vi "Calibration(Z).vi"(7 "Load calibration data":bool, 8 "error in (no error)":errorcluster, 9 "Save calibration data":bool, 10 "Done Button":bool, 11 "Acceleration [g]| Voltage [V]":dbl[][](array[numeric])=[[1.0, 2.02], [3.0, 3.3], [-3.0, 0.25], [0.0, 1.7]]) -> (0 "error out":errorcluster, 2 "Interpolation method":T1(ring), 3 "Distance [cm]| Voltage [V]":dbl[][](array[numeric])=[[1.0, 2.02], [3.0, 3.3], [-3.0, 0.25], [0.0, 1.7]])   [LabVIEW 2025]
uses:
  <vilib>/Utility/file.llb/Write To Spreadsheet File (DBL).vi
  <vilib>/Utility/file.llb/Read From Spreadsheet File (DBL).vi
  <vilib>/gmath/NI_Gmath.lvlib
panel:
  in  "method":T1(ring)=enum."linear"
  in  "Refresh Button":bool
  out "Transfer function":cluster{"yi":dbl[], "xi used":dbl[]}[](graph)=[{"yi"=[2.02, 3.3, 0.25, 1.7], "xi used"=[1.0, 3.0, -3.0, 0.0]}, {"yi"=[0.25, 0.2953125, 0.340625, 0.38593750000000004, 0.43125, 0.47656250000000006, 0.5218750000000001, 0.5671875000000001, 0.6125, 0.6578125, 0.703125, 0.7484375, 0.79375, 0.8390624999999999, 0.8843749999999999, 0.9296875, 0.975, 1.0203125, 1.065625, 1.1109375, 1.15625, 1.2015625, 1.246875, 1.2921874999999998, 1.3375, 1.3828125, 1.4281249999999999, 1.4734374999999997, 1.5187499999999998, 1.5640625, 1.609375, 1.6546875, 1.7, 1.71, 1.7199999999999998, 1.7299999999999998, 1.7399999999999998, 1.7499999999999998, 1.7599999999999998, 1.7699999999999998, 1.7799999999999998, 1.7899999999999998, 1.7999999999999998, 1.8099999999999998, 1.8199999999999998, 1.8299999999999998, 1.8399999999999999, 1.8499999999999999, 1.8599999999999999, 1.8699999999999999, 1.88, 1.89, 1.9, 1.91, 1.92, 1.93, 1.94, 1.95, 1.96, 1.97, 1.98, 1.99, 2.0, 2.01, 2.02, 2.0599999999999996, 2.0999999999999996, 2.1399999999999997, 2.1799999999999997, 2.2199999999999998, 2.26, 2.3, 2.34, 2.38, 2.42, 2.46, 2.5, 2.54, 2.58, 2.62, 2.66, 2.7, 2.74, 2.7800000000000002, 2.8200000000000003, 2.8600000000000003, 2.9000000000000004, 2.9400000000000004, 2.98, 3.0199999999999996, 3.0599999999999996, 3.0999999999999996, 3.1399999999999997, 3.1799999999999997, 3.2199999999999998, 3.26, 3.3], "xi used"=[-3.0, -2.90625, -2.8125, -2.71875, -2.625, -2.53125, -2.4375, -2.34375, -2.25, -2.15625, -2.0625, -1.96875, -1.8750000000000002, -1.7812500000000002, -1.6875000000000002, -1.59375, -1.5, -1.40625, -1.3125, -1.2187500000000004, -1.125, -1.0312499999999996, -0.9375, -0.8437500000000003, -0.75, -0.6562499999999998, -0.5625000000000002, -0.4687500000000006, -0.37500000000000033, -0.2812500000000001, -0.18749999999999983, -0.09374999999999958, 0.0, 0.03125000000000003, 0.06249999999999917, 0.0937499999999992, 0.12499999999999922, 0.15624999999999925, 0.18749999999999928, 0.2187499999999993, 0.24999999999999933, 0.28124999999999933, 0.3124999999999994, 0.34374999999999944, 0.37499999999999944, 0.40624999999999944, 0.4374999999999995, 0.46874999999999956, 0.49999999999999956, 0.5312499999999996, 0.5624999999999996, 0.5937499999999996, 0.6249999999999997, 0.6562499999999998, 0.6874999999999998, 0.7187499999999998, 0.7499999999999998, 0.7812499999999998, 0.8124999999999998, 0.8437499999999998, 0.8749999999999999, 0.90625, 0.9375, 0.9687499999999993, 1.0, 1.0625, 1.125, 1.1875, 1.25, 1.3125, 1.375, 1.4375, 1.5, 1.5625, 1.625, 1.6875, 1.75, 1.8125, 1.875, 1.9375, 2.0, 2.0625, 2.125, 2.1875, 2.25, 2.3125, 2.375, 2.4375, 2.5, 2.5625, 2.625, 2.6875, 2.75, 2.8125, 2.875, 2.9375, 3.0]}]
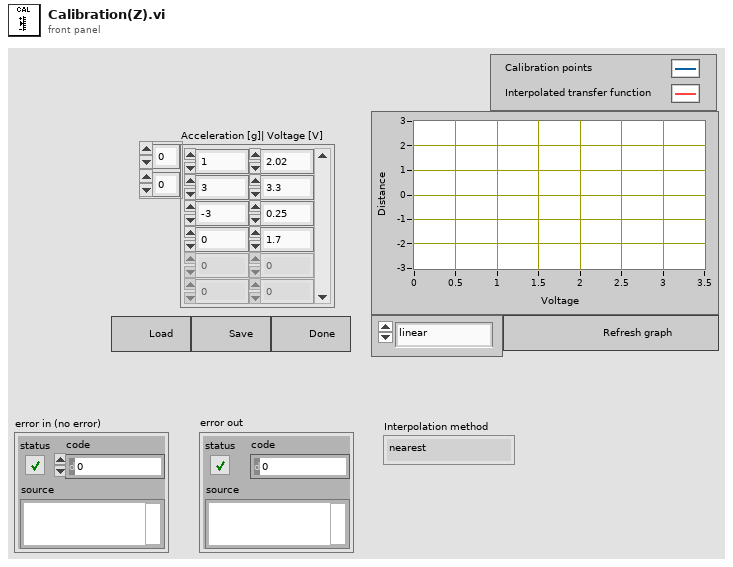
[diagram p1: front panel]
types:
  T1 = enum16{"nearest", "linear", "spline", "cubic Hermite", "Lagrange"}
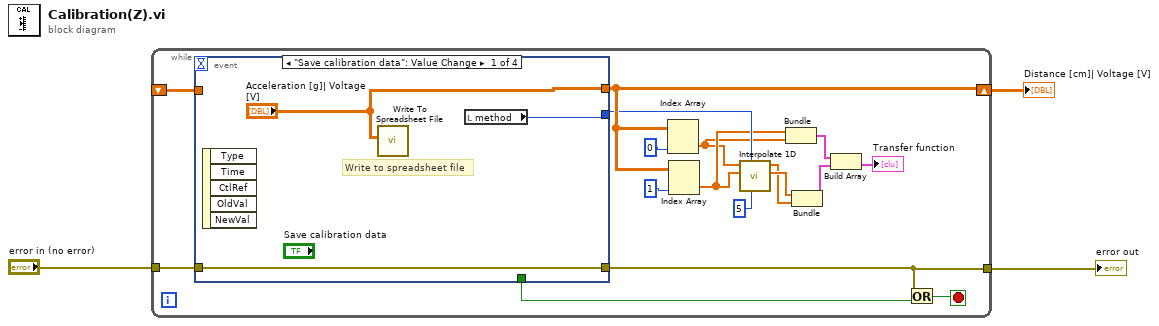
[diagram p0: block diagram]
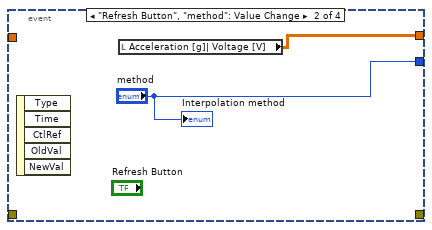
[diagram p2: hidden frame]
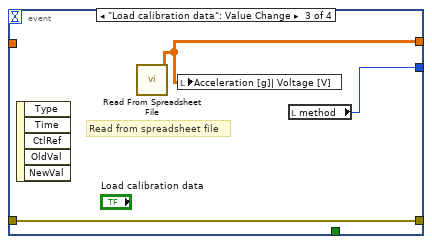
[diagram p3: hidden frame]
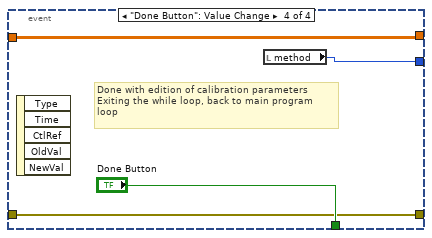
[diagram p4: hidden frame]
diagram:
  n1 = while {
    tunnel: "error in (no error)" -> [w19]
    tunnel: [w18] -> w3
    shift-right: [w13] -> w1
    shift-left: _ -> [w20]
    stop <- w16 stop-if-true
    n2 = event shown="[0] \"Save calibration data\": Value Change" {
      selector: _ -> [_ _ _ _]
      dyn-events: _ -> [_ _ _ _]
      timeout: _ -> [_ _ _ _]
      tunnel: w20 -> [_ _ _ w32]
      tunnel: ["Acceleration [g]| Voltage [V]" w25 w27 w32] -> w13
      tunnel: [_ _ _ "Done Button"] -> w17
      tunnel: w19 -> [w23 _ w28 w30]
      tunnel: [w23 _ w28 w30] -> w18
      tunnel: [w21 "method" w26 w29] -> w8
      event "Save calibration data": Value Change {
        # "Write to spreadsheet file"
        n3 = event-data() -> ()  [unwired: 1 in, 5 out]
        n4 = call-poly <vilib>:"Write To Spreadsheet File.vi"("2D data"="Acceleration [g]| Voltage [V]") -> ()  [unwired: 7 in, 1 out]
        n5 = local read "method"() -> (w21:T1)
      }
      event "Refresh Button", "method": Value Change {
        n6 = event-data() -> ()  [unwired: 1 in, 5 out]
        n7 = local read "Acceleration [g]| Voltage [V]"() -> (w25:dbl[][])
        "Interpolation method" <- "method"
      }
      event "Load calibration data": Value Change {
        # "Read from spreadsheet file"
        n8 = event-data() -> ()  [unwired: 1 in, 5 out]
        n9 = call-poly <vilib>:"Read From Spreadsheet File.vi"() -> ("all rows"=w27:dbl[][])  [unwired: 7 in, 4 out]
        n10 = local write "Acceleration [g]| Voltage [V]"(w27) -> ()
        n11 = local read "method"() -> (w26:T1)
      }
      event "Done Button": Value Change {
        # "Done with edition of calibration parameters\nExiting the while loop, back to main program \nloop"
        n12 = event-data() -> ()  [unwired: 1 in, 5 out]
        n13 = local read "method"() -> (w29:T1)
      }
    }
    n14 = Index Array(array=w13, index (col)=0 ("disabled index (col)")) -> (element=w6:dbl[])  [unwired: 1 in]
    n15 = Index Array(array=w13, index (col)=1 ("disabled index (col)")) -> (element=w7:dbl[])  [unwired: 1 in]
    n16 = call <vilib>:"Interpolate 1D.vi"("ntimes"=5, "method"=w8, "X"=w7, "Y"=w6) -> ("xi used"=w5:dbl[], "yi"=w4:dbl[])  [unwired: 5 in, 1 out]
    n17 = Bundle("all rows"=w7, "all rows"=w6) -> (w11:cluster{"all rows":dbl[], "all rows":dbl[]})  [unwired: 1 in]
    n18 = Bundle("xi used"=w5, "yi"=w4) -> (w10:cluster{"xi used":dbl[], "yi":dbl[]})  [unwired: 1 in]
    n19 = Build Array(w11, w10) -> (→"Transfer function":cluster{"xi used":dbl[], "yi":dbl[]}[])
    n20 = Or(x=w18, y=w17) -> (x .or. y?=w16:bool)
  }
  "error out" <- w3
  "Distance [cm]| Voltage [V]" <- w1
